vi "SR830 set sin out voltage.vi"(8 "error in (no error)":errorcluster, 10 "voltage":dbl[unit], 11 "VISA resource name":refnum<visa-resource-name>) -> (0 "error out":errorcluster, 3 "VISA resource name out":refnum<visa-resource-name>)   [LabVIEW 2009, in "SR830.lvlib"]
doc: "Sets the voltage of the SINE OUT output of the lock-in amplifier."
uses:
  SR830.lvlib
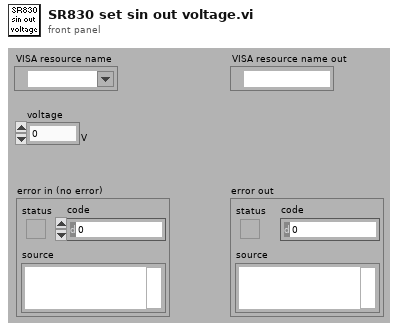
[diagram p1: front panel]
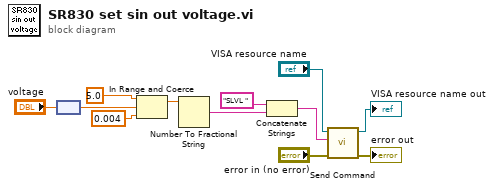
[diagram p0: block diagram]
diagram:
  n1 = node("voltage") -> (w6:dbl)
  n2 = In Range and Coerce(upper limit=5.0, x=w6, lower limit=0.004) -> (coerced(x)=w12:dbl)  [unwired: 1 out]
  n3 = Number To Fractional String(number=w12) -> (F-format string=w8:string)  [unwired: 3 out]
  n4 = Concatenate Strings("SLVL " ("write buffer"), w8) -> (w4:string)
  n5 = call "Send Command.vi"("error in (no error)"="error in (no error)", "write buffer"=w4, "VISA resource name"="VISA resource name") -> ("error out"=→"error out":errorcluster, "VISA resource name out"=→"VISA resource name out":refnum<visa-resource-name>)  [unwired: 7 in]
